vi "pasco_test_vi.vi"(2 "Boolean":bool) -> (0 "pasco_point_slider":dbl)   [LabVIEW 2011]
uses:
  Robot Global Data.vi
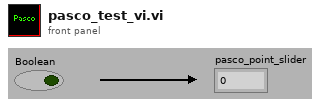
[diagram p1: front panel]
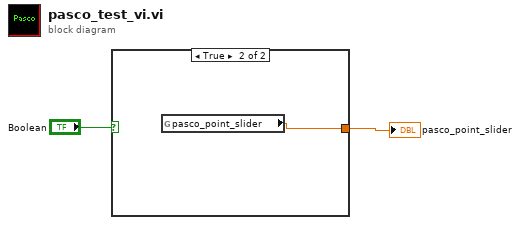
[diagram p0: block diagram]
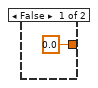
[diagram p2: hidden frame]
diagram:
  n1 = case shown="True" "Boolean" {
    tunnel: [0.0 ("pasco_point_slider") w4] -> w1
    frame False {
    }
    frame True {
      n2 = global read "Robot Global Data.vi" "pasco_point_slider"() -> (w4:dbl)
    }
  }
  "pasco_point_slider" <- w1
